vi "Fetch Rx Data (CDB WDT).vi"(0 "Register Bus":T1, 2 "vertical range [Vpp]":dbl=2.0 format="%#_6p", 5 "number of samples":u32=8196, 9 "timeout [s]":dbl=10.0, 11 "error in":errorcluster, 12 "sample rate [S/s]":dbl=130000000.0 format="%#_6p", 13 "leading samples to trim":i32) -> (4 "Register Bus (out)":T1, 6 "Waveform (CDB WDT)":waveform(cdb), 15 "error out":errorcluster)   [LabVIEW 2017]
doc: "Fetch Rx data from the device. It's required to call <b>Configure Stream</b> and <b>Initiate Stream</b> before calling this VI."
uses:
  <instrlib>/_niInstr/Register Bus/v0/Host/Public/Register Bus Session.ctl
  <instrlib>/_niInstr/Register Bus/v0/Host/Private/Session Data.ctl
  Rx FPGA VI Reference.ctl
  <vilib>/rvi/errors/niLvFpgaAdjustHostInterfaceError.vi
  <vilib>/rvi/interface/nirviMethod/nirviMethod.xnode
  <instrlib>/_niInstr/Register Bus/v0/Host/niInstr Register Bus v0 Host.lvlib
  <vilib>/FPGAPlugInAG/Dynamic/niLvFpga_ReadFifo_Dynamic.vi
  <vilib>/rvi/errors/niLvFpgaMergeErrorWithErrorCode.vi
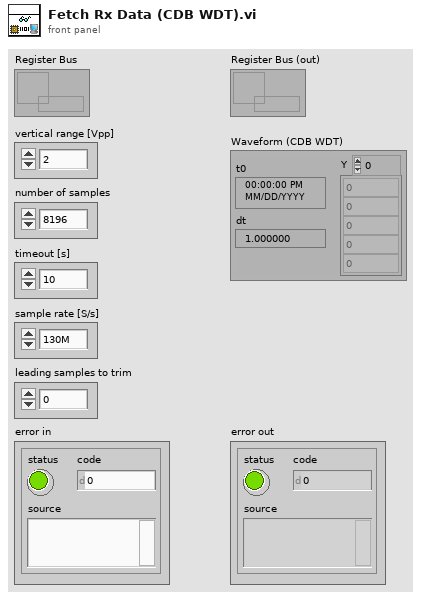
[diagram p1: front panel]
types:
  T1 = typedef "niInstr Register Bus v0 Host.lvlib/Register Bus Session.ctl" = refnum<queue>
  T2 = typedef "Rx FPGA VI Reference.ctl" = refnum<k20>
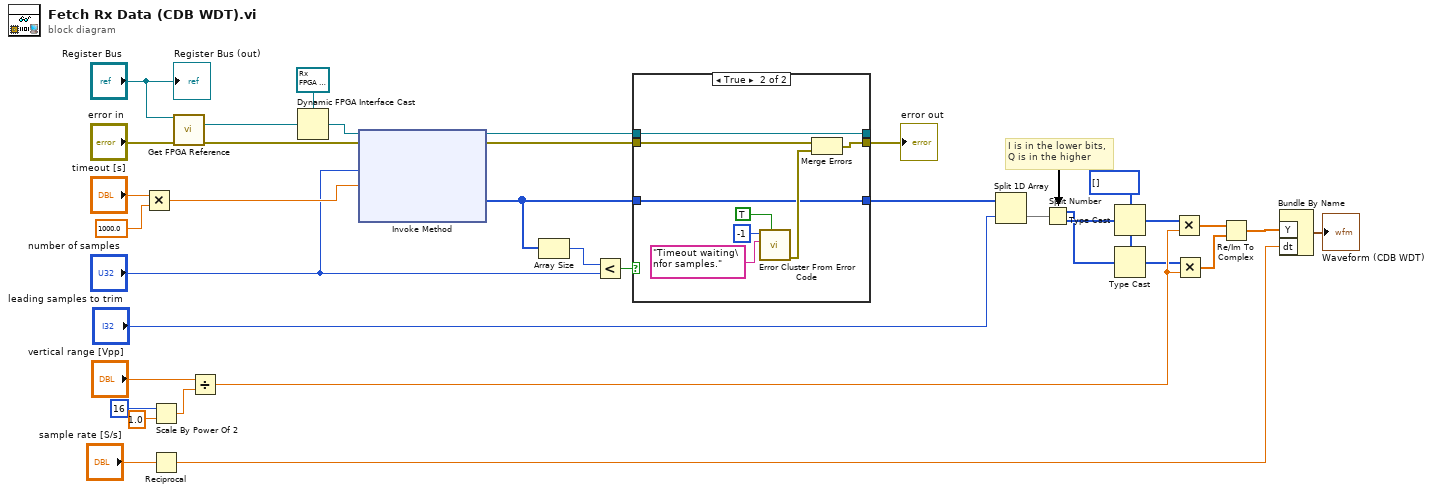
[diagram p0: block diagram]
diagram:
  w12 = i16[] []
  # "I is in the lower bits,\nQ is in the higher"
  n1 = Multiply(x="timeout [s]", y=1000.0) -> (x*y=w26:dbl)
  n2 = Scale By Power Of 2(n=i16 16 ("ADC Resolution (bits)"), x=1.0) -> (x*2^n=w15:dbl)
  n3 = Reciprocal(x="sample rate [S/s]") -> (1/x=w19:dbl)
  n4 = call <instrlib>:"Get FPGA Reference.vi"("session in"="Register Bus", "error in"="error in") -> ("fpga ref"=w33:refnum<k20>, "error out"=w32:errorcluster)  [unwired: 11 in, 1 out]
  n5 = Divide(x="vertical range [Vpp]", y=w15) -> (x/y=w14:dbl)
  n6 = Dynamic FPGA Interface Cast(Session In=T2 refnum ("Type"), Type=w33) -> (Session Out=w31:T2)
  n7 = xnode "Invoke Method"("FPGA VI Reference In"=w31, "error in"=w32, "Number of Elements"="number of samples", "Timeout (ms)"=w26) -> ("FPGA VI Reference Out"=w29:T2, "error out"=w30:errorcluster, "Data"=w4:u32[])  [unwired: 1 out]
  n8 = Array Size(array=w4) -> (size(s)=w3:i32)
  n9 = Less?(x=w3, y="number of samples") -> (x < y?=w24:bool)
  n10 = case shown="True" w24 {
    tunnel: w29 -> [w38 w46]
    tunnel: w30 -> [w37 w43]
    tunnel: [w38 w46] -> _
    tunnel: [w37 w42] -> w22
    tunnel: [w36 w39] -> w2
    tunnel: w4 -> [w36 w39]
    frame False {
    }
    frame True {
      n11 = call <vilib>:"Error Cluster From Error Code.vi"("show call chain? (False)"=TRUE, "error message (\"\")"="Timeout waiting\nfor samples." ("error message (\"\")"), "error code (0)"=-1) -> ("error out"=w41:errorcluster)  [unwired: 6 in]
      n12 = Merge Errors(w43, w41) -> (w42:errorcluster)
    }
  }
  "error out" <- w22
  n13 = Split 1D Array(array=w2, index="leading samples to trim") -> (second subarray=w11:u32[])  [unwired: 1 out]
  n14 = Split Number(x=w11) -> (hi(x)=w5:u16[], lo(x)=w6:u16[])
  n15 = Type Cast(type=w12, x=w6) -> (*(type *) &x=w10:i16[])
  n16 = Type Cast(type=w12, x=w5) -> (*(type *) &x=w9:i16[])
  n17 = Multiply(x=w10, y=w14) -> (x*y=w8:dbl[])
  n18 = Multiply(x=w9, y=w14) -> (x*y=w7:dbl[])
  n19 = Re/Im To Complex(1:w7, 2:w8) -> (0:w1:cdb[])
  n20 = Bundle By Name("Y"=w1, "dt"=w19) -> (→"Waveform (CDB WDT)":waveform(cdb))  [unwired: 1 in]
  "Register Bus (out)" <- "Register Bus"
